vi "Control_Carrito.vi"() -> ()   [LabVIEW 2016]
uses:
  <vilib>/Instr/_visa.llb/VISA Configure Serial Port (Instr).vi
panel:
  in  "Suroeste":bool
  in  "Sureste":bool
  in  "Noroeste":bool
  in  "Noreste":bool
  in  "Stop Button":bool
  in  "Velocidad":u8(knob) scale=0.0..255.0
  in  "Paro":bool
  in  "Retroceder":bool
  in  "Giro Horario":bool
  in  "Giro Antihorario":bool
  in  "Avanzar":bool
  in  "VISA resource name":refnum<visa-resource-name>
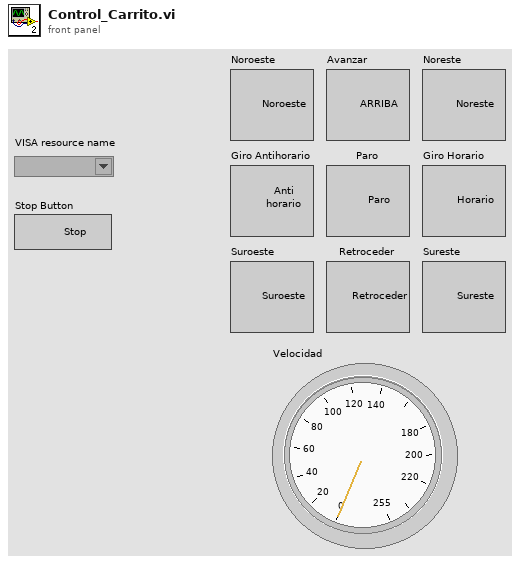
[diagram p1: front panel]
types:
  T1 = cluster{"baud rate (9600)":u32, "data bits (8)":u16, "parity (0:none)":u16, "error in (no error)":errorcluster, "stop bits (10: 1 bit)":u16, "flow control (0:none)":u16}
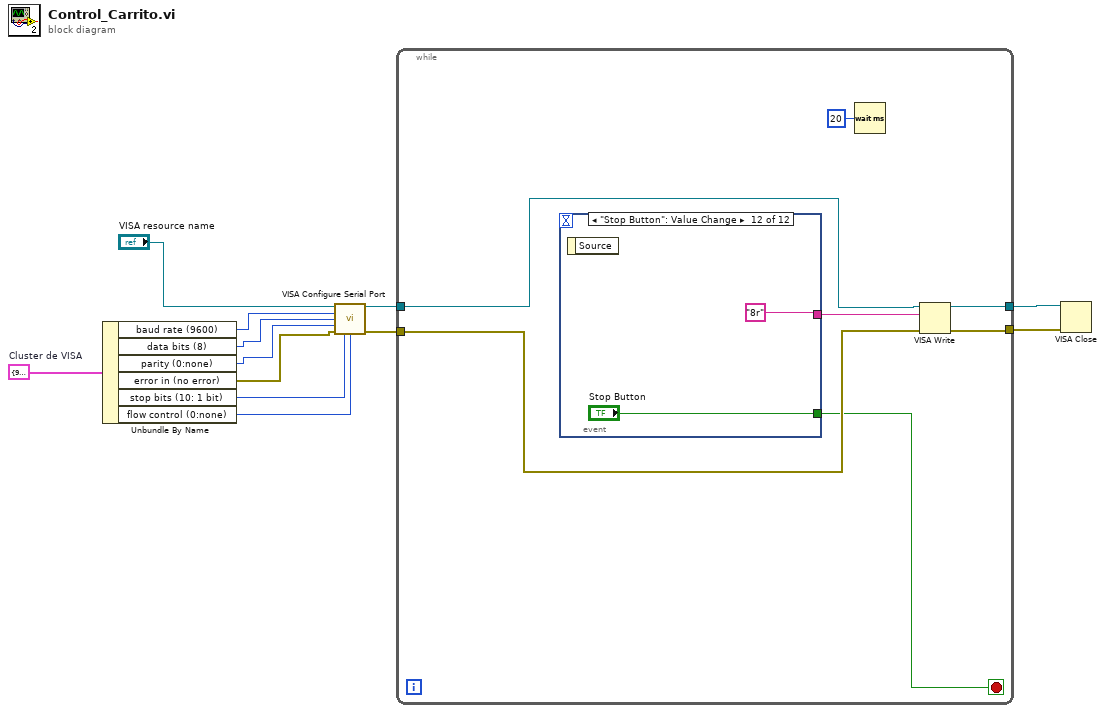
[diagram p0: block diagram]
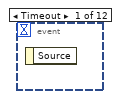
[diagram p2: hidden frame]
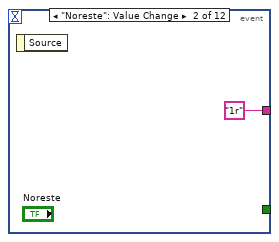
[diagram p3: hidden frame]
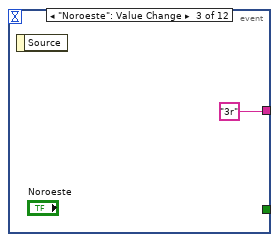
[diagram p4: hidden frame]
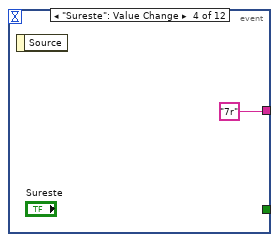
[diagram p5: hidden frame]
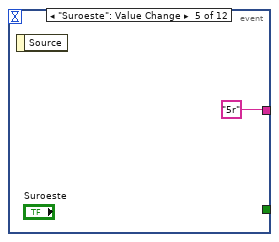
[diagram p6: hidden frame]
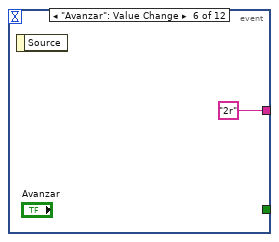
[diagram p7: hidden frame]
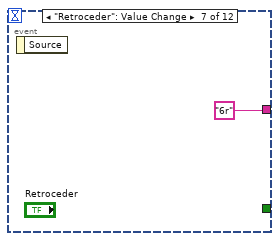
[diagram p8: hidden frame]
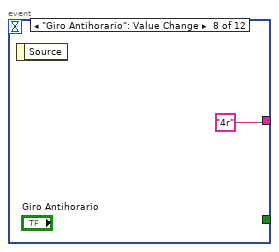
[diagram p9: hidden frame]
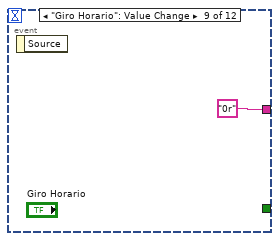
[diagram p10: hidden frame]
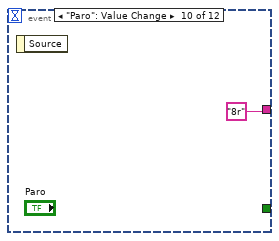
[diagram p11: hidden frame]
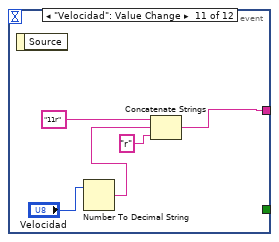
[diagram p12: hidden frame]
diagram:
  w11 = T1 {"baud rate (9600)"=9600, "data bits (8)"=8, "parity (0:none)"=0, "error in (no error)"={"status"=FALSE, "code"=0, "source"=""}, "stop bits (10: 1 bit)"=10, "flow control (0:none)"=0}  # Cluster de VISA
  n1 = Unbundle By Name(w11) -> ("baud rate (9600)"=w10:u32, "data bits (8)"=w8:u16, "parity (0:none)"=w7:u16, "error in (no error)"=w6:errorcluster, "stop bits (10: 1 bit)"=w5:u16, "flow control (0:none)"=w4:u16)
  n2 = call-poly "VISA Configure Serial Port"("VISA resource name"="VISA resource name", "baud rate (9600)"=w10, "data bits (8)"=w8, "parity (0:none)"=w7, "error in (no error)"=w6, "stop bits (10: 1 bit)"=w5, "flow control (0:none)"=w4) -> ("VISA resource name out"=w9:refnum<visa-resource-name>, "error out"=w3:errorcluster)  [unwired: 7 in]
  n3 = while {
    tunnel: w9 -> [w16]
    tunnel: w3 -> [w17]
    tunnel: [w14] -> w2
    tunnel: [w15] -> w1
    stop <- w13 stop-if-true
    n4 = event shown="[11] \"Stop Button\": Value Change" {
      selector: _ -> [_ _ _ _ _ _ _ _ _ _ _ _]
      dyn-events: _ -> [_ _ _ _ _ _ _ _ _ _ _ _]
      timeout: _ -> [_ _ _ _ _ _ _ _ _ _ _ _]
      tunnel: [_ "1r" "3r" "7r" "5r" "2r" "6r" "4r" "0r" "8r" w29 "8r"] -> w18
      tunnel: [_ _ _ _ _ _ _ _ _ _ _ "Stop Button"] -> w13
      event Timeout {
        n5 = event-data() -> ()  [unwired: 1 in, 1 out]
      }
      event "Noreste": Value Change {
        n6 = event-data() -> ()  [unwired: 1 in, 1 out]
      }
      event "Noroeste": Value Change {
        n7 = event-data() -> ()  [unwired: 1 in, 1 out]
      }
      event "Sureste": Value Change {
        n8 = event-data() -> ()  [unwired: 1 in, 1 out]
      }
      event "Suroeste": Value Change {
        n9 = event-data() -> ()  [unwired: 1 in, 1 out]
      }
      event "Avanzar": Value Change {
        n10 = event-data() -> ()  [unwired: 1 in, 1 out]
      }
      event "Retroceder": Value Change {
        n11 = event-data() -> ()  [unwired: 1 in, 1 out]
      }
      event "Giro Antihorario": Value Change {
        n12 = event-data() -> ()  [unwired: 1 in, 1 out]
      }
      event "Giro Horario": Value Change {
        n13 = event-data() -> ()  [unwired: 1 in, 1 out]
      }
      event "Paro": Value Change {
        n14 = event-data() -> ()  [unwired: 1 in, 1 out]
      }
      event "Velocidad": Value Change {
        n15 = event-data() -> ()  [unwired: 1 in, 1 out]
        n16 = Number To Decimal String(number="Velocidad") -> (decimal integer string=w31:string)  [unwired: 1 in]
        n17 = Concatenate Strings("11r", w31, "r" ("string")) -> (w29:string)
      }
      event "Stop Button": Value Change {
        n18 = event-data() -> ()  [unwired: 1 in, 1 out]
      }
    }
    n19 = Wait (ms)(milliseconds to wait=u32 20) -> ()  [unwired: 1 out]
    n20 = VISA Write(VISA resource name=w16, write buffer=w18, error in (no error)=w17) -> (VISA resource name out=w15:refnum<visa-resource-name>, error out=w14:errorcluster)  [unwired: 1 out]
  }
  n21 = VISA Close(VISA resource name=w1, error in (no error)=w2) -> ()  [unwired: 1 out]
